vi "BenchC2.vi"() -> ()   [LabVIEW 2016]
uses:
  x64/Debug/BERTTA.dll
panel:
  out "element":bool
  out "Started:":string
  in  "SHUTDOWN":bool
  in  "MASTER CONTROL":bool
  in  "Tab Control":T1(tab)
  out "Output File":path caption="selected path"
  in  "Browse folder":path=path "" caption="start path"
  in  "Read Seq":bool
  in  "Save Seq":bool
  in  "Configuration file":path=path "C:/Users/shresplab/Desktop/ArttuConfiguration.lvm" caption="Filename"
  in  "OK Button 2":bool
  out "Boolean":bool
  in  "User (initials)":string
  in  "Project name":string
  in  "Description":string
  out "PUMP1":bool
  out "Target amount":dbl
  out "Scale weight":dbl
  out "Amount now":dbl
  out "Flow rate":dbl
  out "Time to target":dbl format="%<%H:%M:%S>t"
  out "Current step":dbl
  out "Target":dbl
  out "Amount now":dbl
  out "Amount now":dbl
  out "Target":dbl
  out "Current step":dbl
  out "Time to target":dbl format="%<%H:%M:%S>t"
  out "Flow rate":dbl
  out "Amount now":dbl
  out "Scale weight":dbl
  out "Target amount":dbl
  out "PUMP2":bool
  out "Sensor OK 6":bool
  out "Sensor OK 5":bool
  out "Sensor OK 4":bool
  out "Sensor OK 3":bool
  in  "OK Button":bool
  in  "Add comment":string
  out "PUMP3":bool
  out "Target amount":dbl
  out "Scale weight":dbl
  out "Amount now":dbl
  out "Flow rate":dbl
  out "Time to target":dbl format="%<%H:%M:%S>t"
  out "Current step":dbl
  out "Target":dbl
  out "Amount now":dbl
  out "Tr":dbl
  out "Tj in":dbl
  out "Tj out":dbl
  out "T set":dbl
  out "Current step":i32
  out "RPM":dbl
  out "Torque 2":dbl
  out "Waveform Chart 5":dynamicdata(graph)
  out "Waveform Chart 6":dynamicdata(graph)
  out "Waveform Chart 7":dynamicdata(graph)
  in  "Tab Control 2":T2(tab)
  out "Waveform Chart 3":dynamicdata(graph)
  out "Waveform Chart 8":dynamicdata(graph)
  out "Waveform Chart 11":dynamicdata(graph)
  out "Waveform Chart 13":dynamicdata(graph)
  out "Waveform Chart 9":dynamicdata(graph)
  out "Table":string[][](table)=[["14.8.2017 18.06.59", "0,000000", "417,670000", "-0,150000", "1,000000", "22,220000", "23,366837", "23,574959", "23,985852", "23,690000", "240,000000", "4,000000", "0,000000", "397,000000", "-397,000000", "1,000000"], ["14.8.2017 18.07.06", "0,000000", "417,640000", "-0,120000", "1,000000", "22,220000", "23,763115", "23,906257", "23,985694", "23,680000", "240,000000", "4,000000", "0,000000", "397,000000", "-397,000000", "1,000000"], ["14.8.2017 18.07.13", "0,000000", "417,640000", "-0,120000", "1,000000", "22,220000", "23,965922", "24,013440", "23,984906", "23,670000", "240,000000", "4,100000", "3,000000", "397,000000", "-397,000000", "1,000000"], ["14.8.2017 18.07.21", "0,000000", "417,640000", "-0,120000", "1,000000", "22,220000", "23,943860", "23,900110", "23,987113", "23,670000", "240,000000", "4,000000", "0,000000", "397,000000", "-397,000000", "1,000000"], ["14.8.2017 18.07.28", "0,000000", "417,640000", "-0,120000", "1,000000", "22,220000", "23,736328", "23,600018", "23,989004", "23,660000", "240,000000", "4,000000", "0,000000", "397,000000", "-397,000000", "1,000000"], ["14.8.2017 18.07.36", "0,000000", "417,640000", "-0,120000", "1,000000", "22,220000", "23,480910", "23,324538", "23,991053", "23,660000", "240,000000", "4,000000", "0,000000", "397,000000", "-397,000000", "1,000000"], ["14.8.2017 18.07.43", "0,000000", "417,640000", "-0,120000", "2,000000", "22,220000", "23,195579", "23,008270", "23,999093", "23,650000", "240,000000", "4,000000", "0,000000", "397,000000", "-397,000000", "1,000000"], ["14.8.2017 18.07.51", "0,000000", "417,650000", "-417,650000", "1,000000", "22,220000", "22,862541", "22,649021", "24,003979", "23,650000", "240,000000", "4,000000", "0,000000", "397,000000", "-397,000000", "2,000000"], ["14.8.2017 18.07.58", "0,000000", "417,640000", "0,010000", "1,000000", "22,220000", "22,541353", "22,354878", "24,005398", "23,650000", "240,000000", "4,000000", "0,000000", "397,000000", "-397,000000", "1,000000"], ["14.8.2017 18.08.06", "0,000000", "417,640000", "0,010000", "1,000000", "22,220000", "22,347931", "22,253738", "24,007605", "23,640000", "240,000000", "4,100000", "0,000000", "397,000000", "-397,000000", "1,000000"], ["14.8.2017 18.08.13", "0,000000", "417,640000", "0,010000", "1,000000", "22,220000", "22,329030", "22,302102", "24,006028", "23,640000", "240,000000", "4,000000", "0,000000", "395,820000", "-395,820000", "1,000000"], ["14.8.2017 18.08.20", "0,000000", "417,640000", "0,010000", "1,000000", "22,220000", "22,466849", "22,511320", "24,002403", "23,630000", "240,000000", "4,000000", "0,000000", "395,830000", "-0,010000", "1,000000"], ["14.8.2017 18.08.28", "0,000000", "417,640000", "0,010000", "1,000000", "22,220000", "22,707062", "22,835101", "24,000984", "23,620000", "240,000000", "4,000000", "0,000000", "395,830000", "-0,010000", "1,000000"], ["14.8.2017 18.08.35", "0,000000", "417,640000", "0,010000", "1,000000", "22,220000", "23,054104", "23,232979", "24,001299", "23,600000", "240,000000", "4,000000", "0,000000", "395,830000", "-0,010000", "1,000000"], ["14.8.2017 18.08.43", "0,000000", "417,640000", "0,010000", "1,000000", "22,220000", "23,412371", "23,522793", "24,002560", "23,590000", "240,000000", "4,000000", "0,000000", "395,820000", "0,000000", "1,000000"], ["14.8.2017 18.08.51", "0,000000", "417,640000", "0,010000", "1,000000", "22,220000", "23,596247", "23,656125", "24,003821", "23,580000", "240,000000", "4,000000", "0,000000", "395,820000", "0,000000", "1,000000"]]
  in  "X scale":i64(slide)=50 scale=0.0..100.0
  in  "Tr/Tj mode selector 2":bool=TRUE
  in  "Tr/Tj mode selector":bool=TRUE
  out "Boolean 4":bool
  out "Boolean 3":bool
  out "Boolean 2":bool
  in  "Reset 6":bool
  in  "Manual/Ramp":bool=TRUE
  in  "Array":dbl[][](array[numeric])=[[20.0, 0.0], [20.0, 0.0], [20.0, 0.0]]
  in  "?":bool
  in  "Time":dbl format="Time to target (min):                %#_g"
  out "Current temp":dbl format="Current temperature (S1):   %#_6g"
  in  "OK Button 3":bool
  out "Sensor OK":bool
  in  "T fail":dbl=20.0 format="Failsafe temperature:              %#_g"
  in  "Setpoint":dbl=20.0 format="Temperature target:                %#_6g"
  out "Waveform Chart":dynamicdata(graph)
  out "T external 2":dbl format="Current temp S2:    %#_g"
  in  "UPDATE TEMP":bool
  out "Led11 5":bool
  out "RPM":dbl format="%_4f"
  out "Led10 3":bool
  out "Led9 3":bool
  out "Led8 3":bool
  out "Led7 3":bool
  out "Led6 3":bool
  out "Led5 3":bool
  out "Led4 3":bool
  out "Led3 3":bool
  out "Led2 3":bool
  out "Led1 3":bool
  in  "PumpSeq 4":dbl[][](array[numeric])=[[0.0, 0.0, 0.0, 0.0, 0.0, 0.0, 0.0, 0.0, 0.0, 0.0], [0.0, 0.0, 0.0, 0.0, 0.0, 0.0, 0.0, 0.0, 0.0, 0.0], [0.0, 0.0, 0.0, 0.0, 0.0, 0.0, 0.0, 0.0, 0.0, 0.0], [0.0, 0.0, 0.0, 0.0, 0.0, 0.0, 0.0, 0.0, 0.0, 0.0], [0.0, 0.0, 0.0, 0.0, 0.0, 0.0, 0.0, 0.0, 0.0, 0.0], [0.0, 0.0, 0.0, 0.0, 0.0, 0.0, 0.0, 0.0, 0.0, 0.0], [0.0, 0.0, 0.0, 0.0, 0.0, 0.0, 0.0, 0.0, 0.0, 0.0], [0.0, 0.0, 0.0, 0.0, 0.0, 0.0, 0.0, 0.0, 0.0, 0.0], [0.0, 0.0, 0.0, 0.0, 0.0, 0.0, 0.0, 0.0, 0.0, 0.0], [0.0, 0.0, 0.0, 0.0, 0.0, 0.0, 0.0, 0.0, 0.0, 0.0]]
  in  "?":bool
  out "Flow rate (g/min)":dbl
  out "Scale reading":dbl
  out "Step amount now":dbl
  in  "Grams / min":dbl
  out "Waveform Chart 14":dynamicdata(graph)
  in  "?":bool
  out "Total amount now":dbl
  out "Led11 4":bool
  in  "Reset 5":bool
  out "Elapsed / step":i32
  out "Time to target":dbl format="%<%H:%M:%S>t"
  in  "OK Button 4":bool
  out "Led11":bool
  out "RPM":dbl format="%_4f"
  out "Led10":bool
  out "Led9":bool
  out "Led8":bool
  out "Led7":bool
  out "Led6":bool
  out "Led5":bool
  out "Led4":bool
  out "Led3":bool
  out "Led2":bool
  out "Led1":bool
  in  "PumpSeq 2":dbl[][](array[numeric])=[[0.0, 0.0, 0.0, 0.0, 0.0, 0.0, 0.0, 0.0, 0.0, 0.0], [0.0, 0.0, 0.0, 0.0, 0.0, 0.0, 0.0, 0.0, 0.0, 0.0], [0.0, 0.0, 0.0, 0.0, 0.0, 0.0, 0.0, 0.0, 0.0, 0.0], [0.0, 0.0, 0.0, 0.0, 0.0, 0.0, 0.0, 0.0, 0.0, 0.0], [0.0, 0.0, 0.0, 0.0, 0.0, 0.0, 0.0, 0.0, 0.0, 0.0], [0.0, 0.0, 0.0, 0.0, 0.0, 0.0, 0.0, 0.0, 0.0, 0.0], [0.0, 0.0, 0.0, 0.0, 0.0, 0.0, 0.0, 0.0, 0.0, 0.0], [0.0, 0.0, 0.0, 0.0, 0.0, 0.0, 0.0, 0.0, 0.0, 0.0], [0.0, 0.0, 0.0, 0.0, 0.0, 0.0, 0.0, 0.0, 0.0, 0.0], [0.0, 0.0, 0.0, 0.0, 0.0, 0.0, 0.0, 0.0, 0.0, 0.0]]
  in  "?":bool
  out "Flow rate (g/min)":dbl
  out "Scale reading":dbl
  out "Step amount now":dbl
  in  "Grams / min":dbl
  out "Waveform Chart 10":dynamicdata(graph)
  in  "?":bool
  out "Total amount now":dbl
  out "Led11":bool
  in  "Reset 3":bool
  out "Elapsed / step":i32
  out "Time to target":dbl format="%<%H:%M:%S>t"
  in  "OK Button 5":bool
  out "Led11 3":bool
  out "RPM":dbl format="%_4f"
  out "Led10 2":bool
  out "Led9 2":bool
  out "Led8 2":bool
  out "Led7 2":bool
  out "Led6 2":bool
  out "Led5 2":bool
  out "Led4 2":bool
  out "Led3 2":bool
  out "Led2 2":bool
  out "Led1 2":bool
  in  "PumpSeq 3":dbl[][](array[numeric])=[[0.0, 0.0, 0.0, 0.0, 0.0, 0.0, 0.0, 0.0, 0.0, 0.0], [0.0, 0.0, 0.0, 0.0, 0.0, 0.0, 0.0, 0.0, 0.0, 0.0], [0.0, 0.0, 0.0, 0.0, 0.0, 0.0, 0.0, 0.0, 0.0, 0.0], [0.0, 0.0, 0.0, 0.0, 0.0, 0.0, 0.0, 0.0, 0.0, 0.0], [0.0, 0.0, 0.0, 0.0, 0.0, 0.0, 0.0, 0.0, 0.0, 0.0], [0.0, 0.0, 0.0, 0.0, 0.0, 0.0, 0.0, 0.0, 0.0, 0.0], [0.0, 0.0, 0.0, 0.0, 0.0, 0.0, 0.0, 0.0, 0.0, 0.0], [0.0, 0.0, 0.0, 0.0, 0.0, 0.0, 0.0, 0.0, 0.0, 0.0], [0.0, 0.0, 0.0, 0.0, 0.0, 0.0, 0.0, 0.0, 0.0, 0.0], [0.0, 0.0, 0.0, 0.0, 0.0, 0.0, 0.0, 0.0, 0.0, 0.0]]
  in  "?":bool
  out "Flow rate (g/min)":dbl
  out "Scale reading":dbl
  out "Step amount now":dbl
  in  "Grams / min":dbl
  out "Waveform Chart 12":dynamicdata(graph)
  in  "?":bool
  out "Total amount now":dbl
  out "Led11 2":bool
  in  "Reset 4":bool
  out "Elapsed / step":i32
  out "Time to target":dbl format="%<%H:%M:%S>t"
  in  "OK Button 6":bool
  in  "?":bool
  in  "Scale port":dbl=5.0
  out "Waveform Chart 15":dynamicdata(graph)
  in  "?":bool
  in  "OK Button 8":bool
  in  "Remote / Manual":bool
  in  "Set RPM":i32
  out "RPM":dbl
  out "Torque":dbl
  out "Waveform Chart 4":dynamicdata(graph)
  in  "OK Button 7":bool
  out "PortDev out":dbl[](array[numeric])
  in  "Save PortDev":bool
  out "PortDev in":dbl[](array[numeric])
  in  "dev1":i32
  in  "dev2":i32
  in  "dev3":i32
  in  "dev4":i32
  in  "dev5":i32
  in  "dev6":i32
  in  "dev8":i32
  in  "port1":i32
  in  "port2":i32
  in  "port3":i32
  in  "port4":i32
  in  "port5":i32
  in  "port6":i32
  in  "port7":i32
  in  "port8":i32
  in  "dev7":i32
  in  "Treshold (T/C)":dbl=0.5
  out "DAQ 9217 (PT100)":errorcluster
  out "Config File":dbl[][](array[numeric])
  in  "Temp Control":tag="cDAQ9188XT-1C3BF2FMod1"
  in  "PAM Control":tag="cDAQ9188XT-1C3BF2FMod7"
  # "Temperature sensor:"
  # "Manual control:"
  # "PUMP & SCALE 1"
  # "STEP"
  # "TOTAL"
  # "PUMP & SCALE 2"
  # "STEP"
  # "TOTAL"
  # "PUMP & SCALE 3"
  # "STEP"
  # "TOTAL"
  # "Temperature control parameter"
  # "Secondary temperature sensor"
  # "Temp target"
  # "Time target"
  # "Grams    /   min"
  # "End of sequence"
  # "Manual control"
  # "Grams    /   min"
  # "End of sequence"
  # "Manual control"
  # "Grams    /   min"
  # "End of sequence"
  # "Manual control"
  # "PAM control"
  # "dev1 and dev2 always to port1 and 2\nport1 = port2 = Lauda\n\ndev3 and dev4 always to port3 and port4\nport3 = port4 = Heidolph"
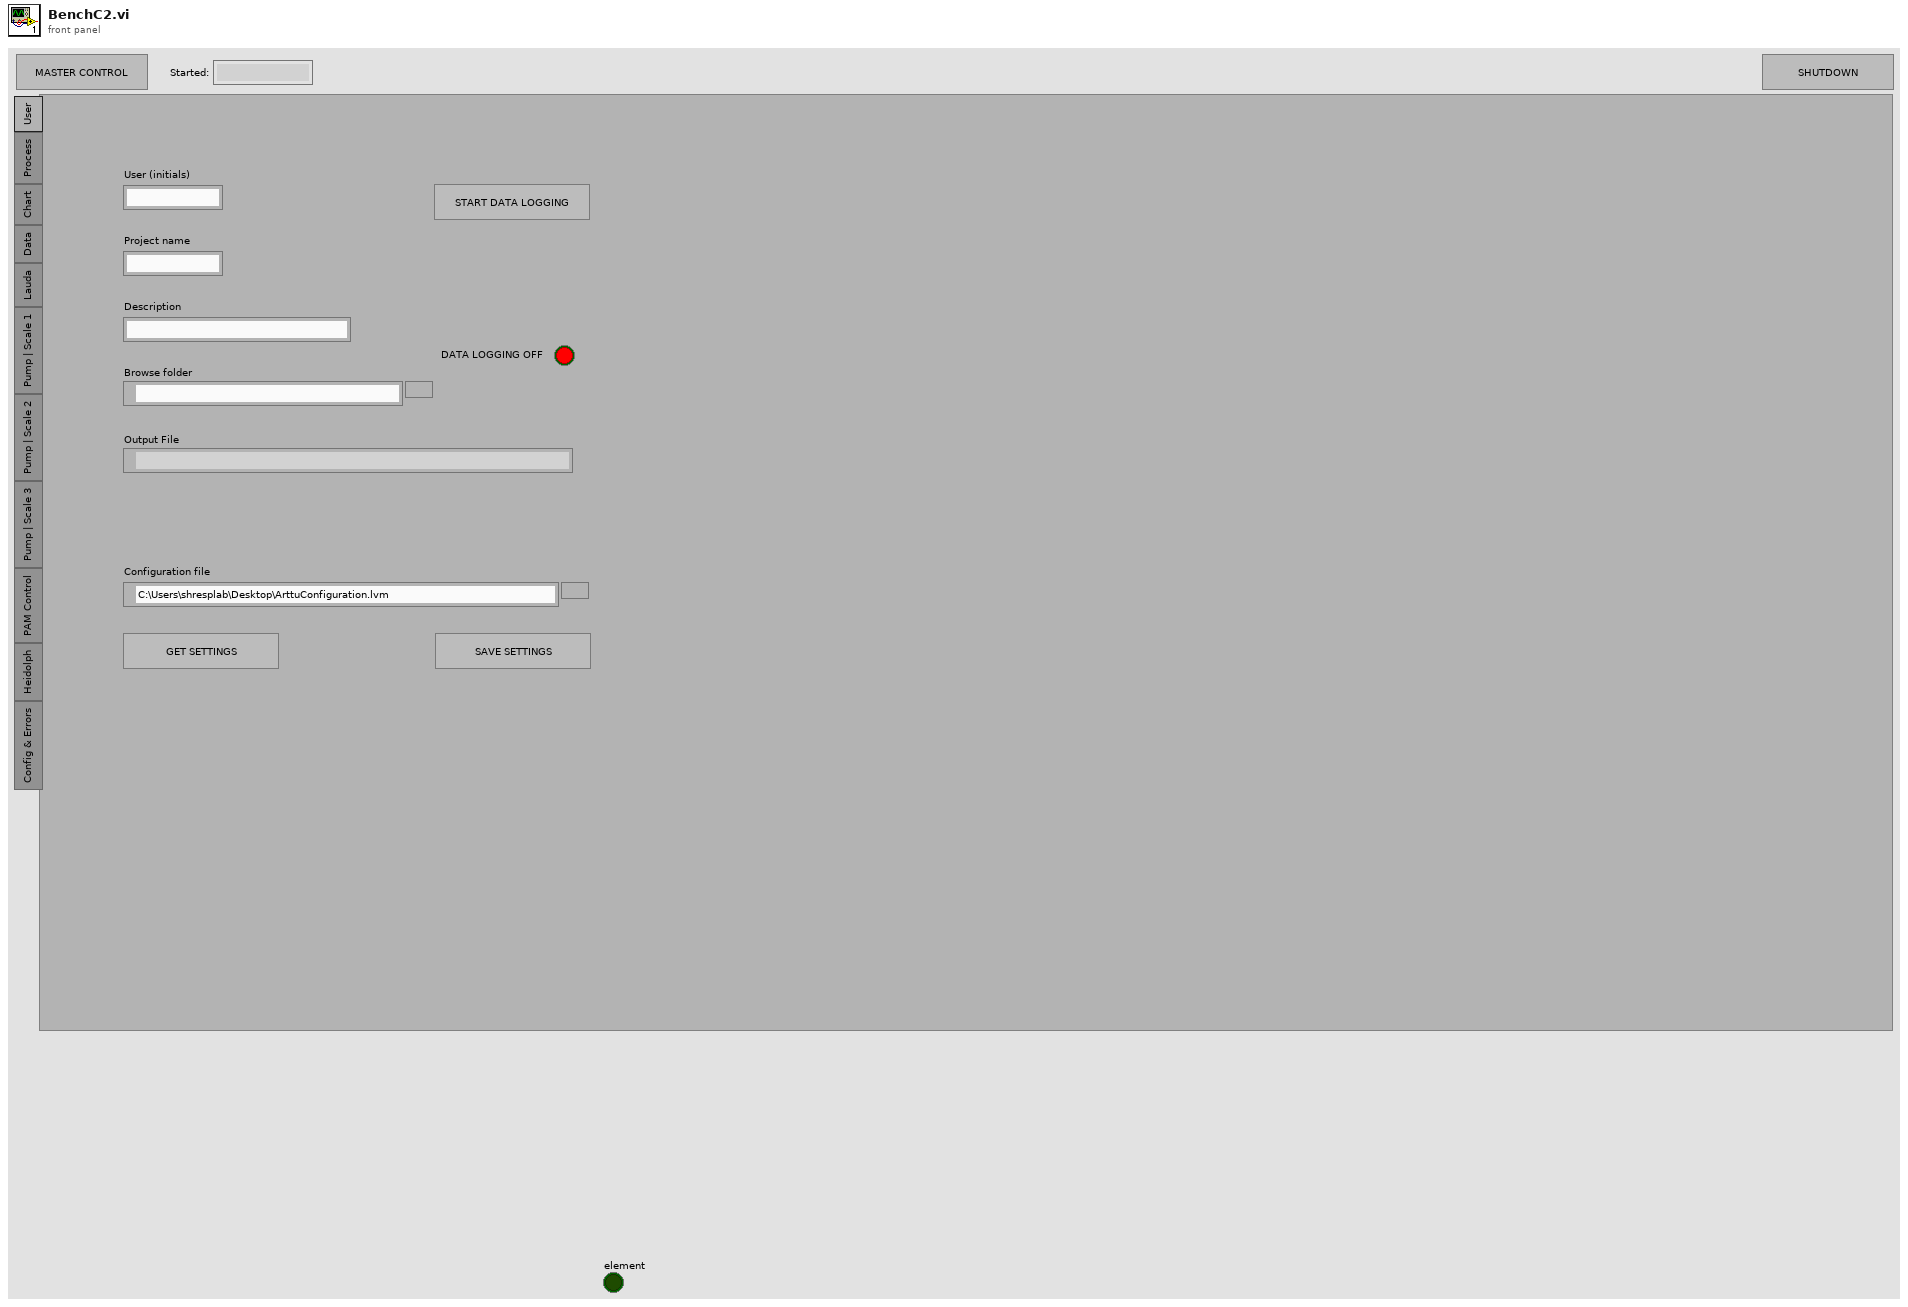
[diagram p1: front panel]
types:
  T1 = enum32{"User", "Process", "Chart", "Data", "Lauda", "Pump | Scale 1", "Pump | Scale 2", "Pump | Scale 3", "PAM Control", "Heidolph", "Config & Errors"}
  T2 = enum32{"Temperatures", "Scale / Pump 1", "Scale / Pump 2", "Scale / Pump 3", "RPM / torque"}
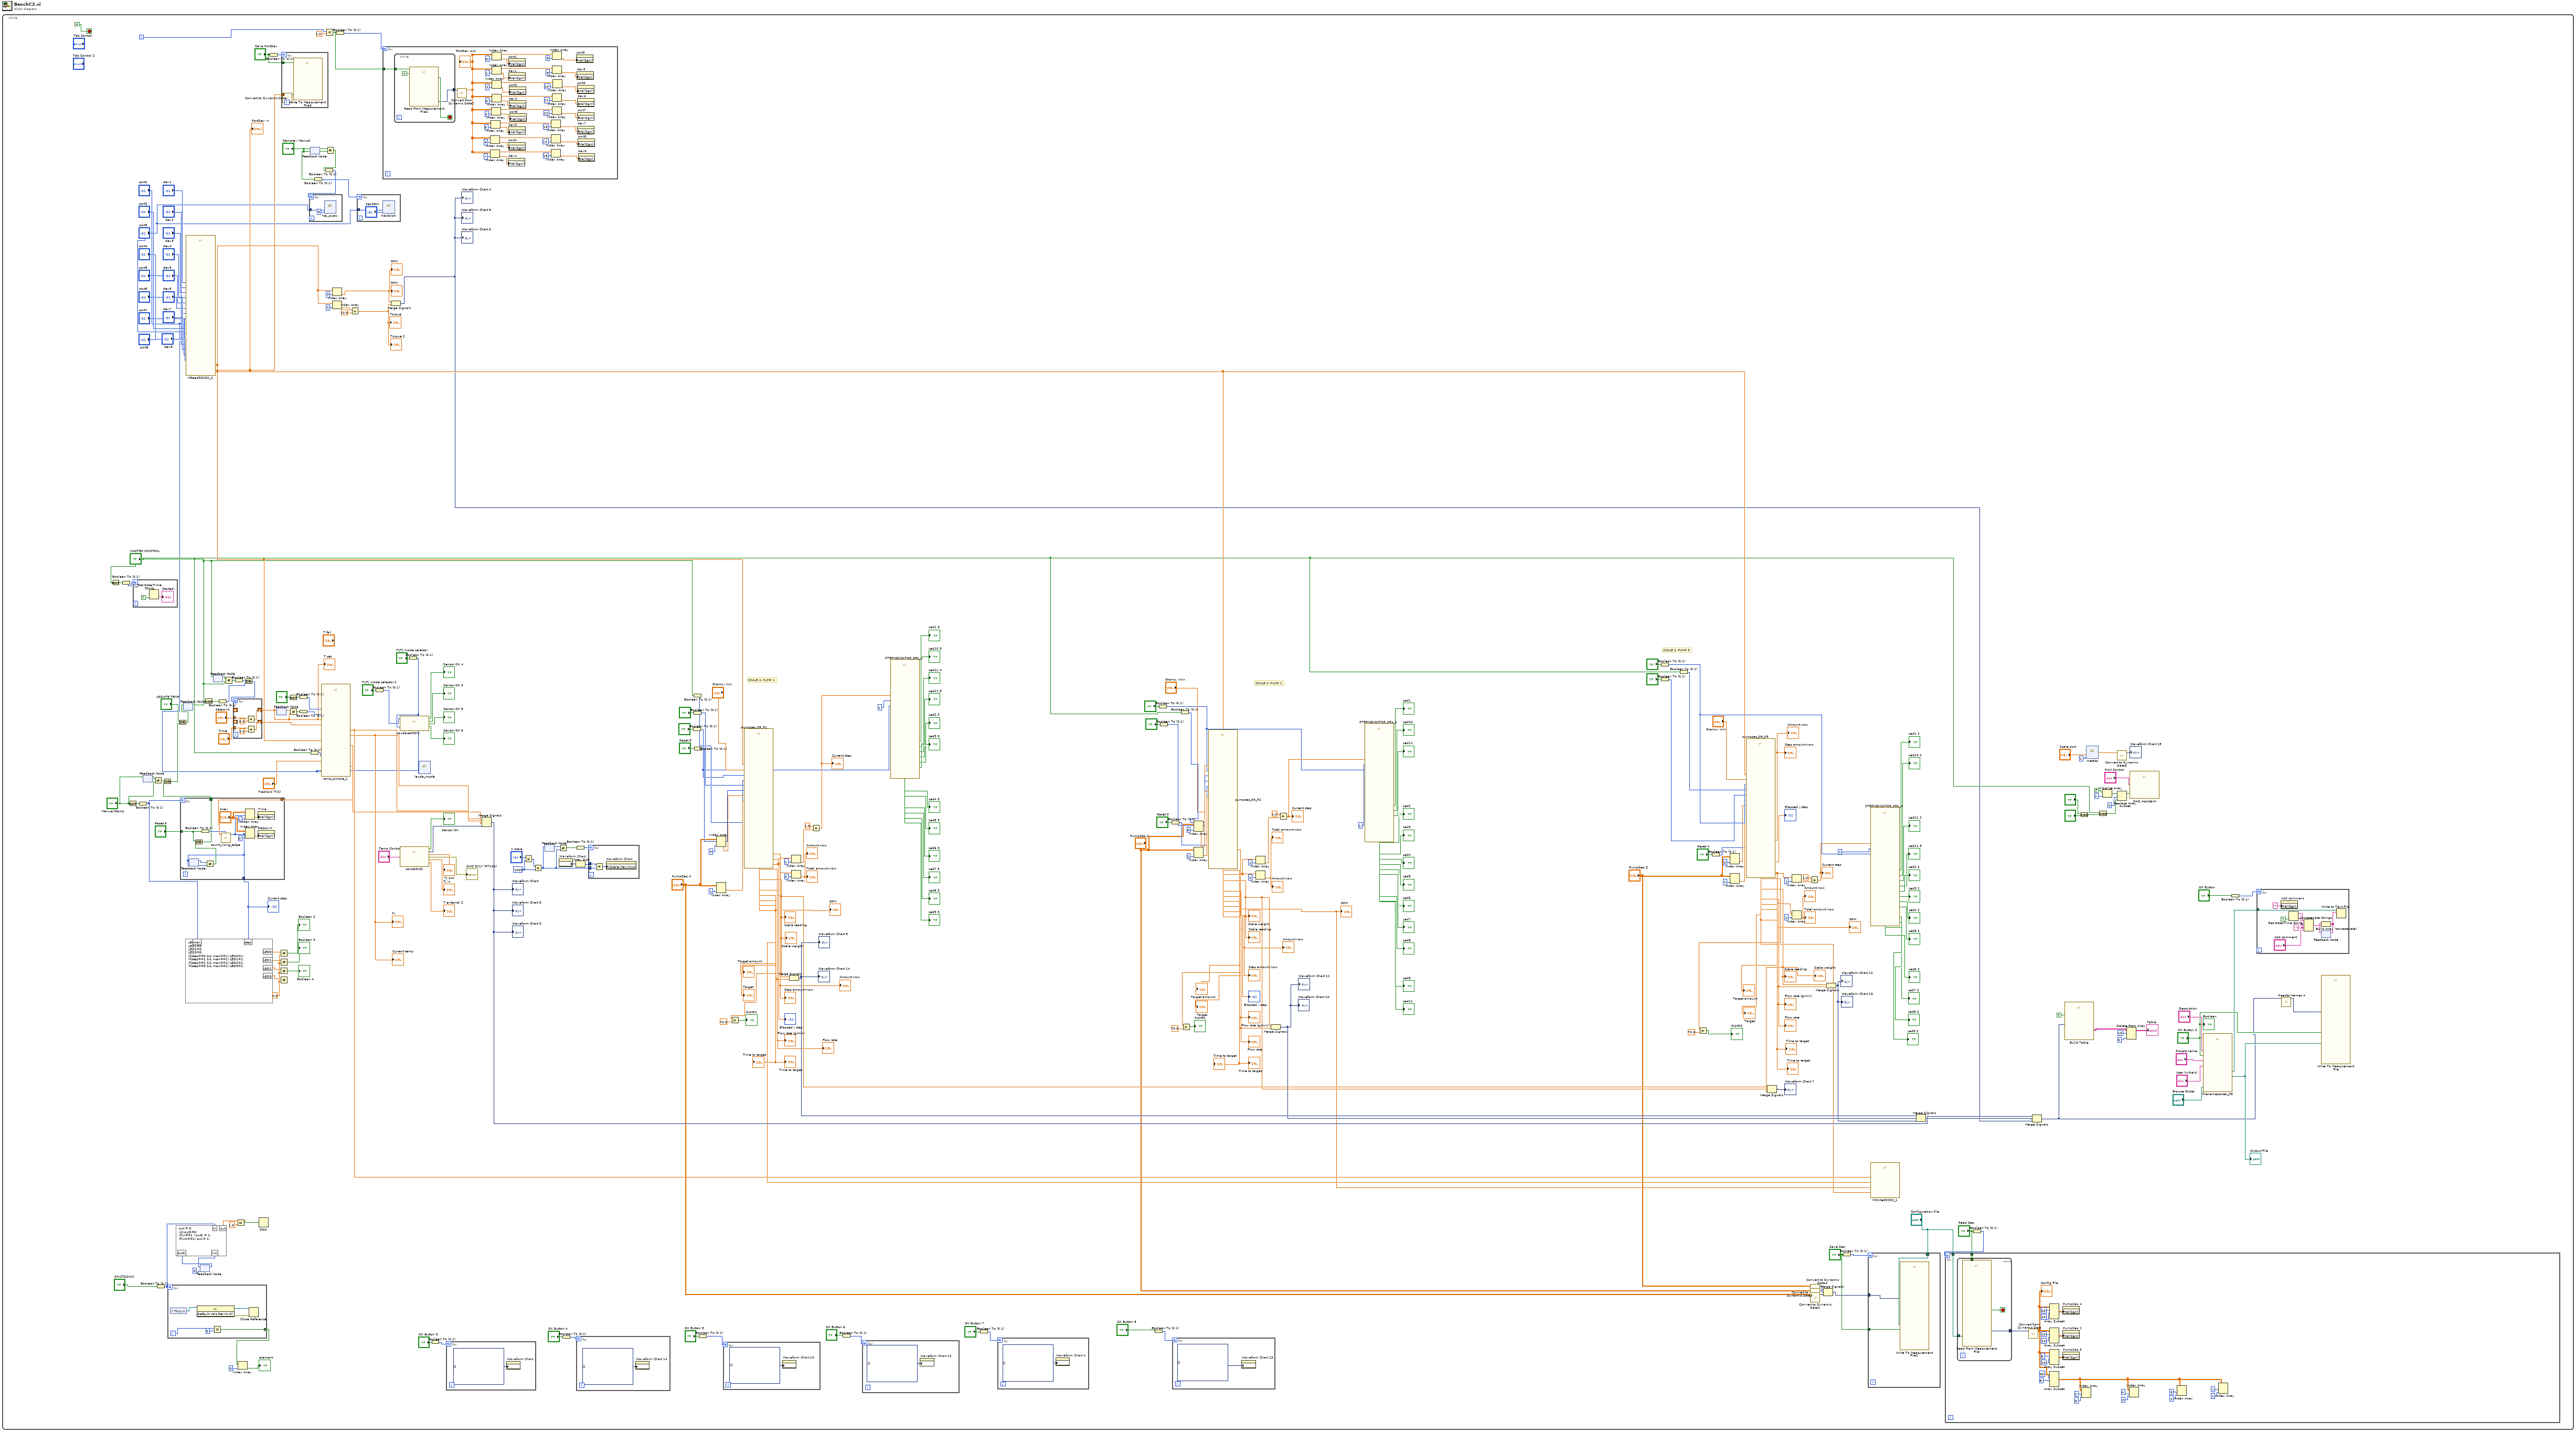
[diagram p0: block diagram]
diagram:
  n1 = while {
    i -> [w75]
    stop <- FALSE stop-if-true
    w6 = i64 1000 ("y")
    w61 = 0.0 ("y")
    # "SCALE & PUMP 1"
    # "SCALE & PUMP 3"
    # "SCALE & PUMP 2"
    n2 = Not(x="MASTER CONTROL") -> (.not. x?=w301:bool)
    n3 = Boolean To (0,1)(Boolean=w301) -> (0, 1=w302:i16)
    n4 = Not(x="Manual/Ramp") -> (.not. x?=w68:bool)
    n5 = for {
      N: w302 -> [_]
      n6 = Get Date/Time String(want seconds? (F)=TRUE) -> (time string=→"Started:":string)  [unwired: 2 in, 1 out]
    }
    n7 = Boolean To (0,1)(Boolean=w68) -> (0, 1=w51:i16)
    n8 = feedback #1() -> (w57:bool)  [unwired: 1 in]
    n9 = feedback-in #1("Manual/Ramp") -> ()
    n10 = Not Equal?(x=w57, y="Manual/Ramp") -> (x != y?=w54:bool)
    n11 = Boolean To (0,1)(Boolean="SHUTDOWN") -> (0, 1=w286:i16)
    n12 = for {
      N: w286 -> [_]
      tunnel: [w421] -> w300 mode=indexing
      i -> [w423]
      n13 = control-ref of="This VI"() -> (w426:refnum<vi>)
      n14 = invoke class="VI" method="Default Vals.Reinit All"(reference=w426) -> (reference out=w424:refnum<vi>, error out=w425:errorcluster)  [unwired: 2 in, 1 out]
      n15 = Greater?(x=w423, y=0) -> (0:w421:bool)
      n16 = Close Reference(reference=w424, error in (no error)=w425) -> ()  [unwired: 1 out]
    }
    n17 = feedback #2() -> (w49:bool)  [unwired: 1 in]
    n18 = call "MReadRS232_2.vi"("port1"="port1", "dev1"="dev1", "port2"="port2", "dev2"="dev2", "port3"="port3", "dev7"="dev7", "dev8"="dev8", "port7"="port7", "port8"="port8", "dev5"="dev5", "port5"="port5", "dev4"="dev4", "dev6"="dev6", "port6"="port6", "port4"="port4", "dev3"="dev3") -> ("output array"=w79:dbl[], "params"=w41:dbl[])  [unwired: 2 in]
    "PortDev in" <- w79
    n19 = feedback #3(0) -> (w284:i32)
    n20 = formula code="out = 0;\nint out2=0;\nif(in==1 ) out2 = 1;\nif(in2==1) out = 1;"("in"=w286, "in2"=w284) -> ("out"=w288:dbl, "out2"=w285:i32)
    n21 = feedback-in #3(w285) -> ()
    n22 = And(x="MASTER CONTROL", y=w49) -> (x .and. y?=w105:bool)
    n23 = feedback #4() -> (w97:bool)  [unwired: 1 in]
    n24 = feedback-in #4("MASTER CONTROL") -> ()
    n25 = Boolean To (0,1)(Boolean=w105) -> (0, 1=w95:i16)
    n26 = Not Equal?(x=w97, y="MASTER CONTROL") -> (x != y?=w96:bool)
    n27 = Boolean To (0,1)(Boolean=w96) -> (0, 1=w94:i16)
    n28 = Equal?(x=w288, y=1.0) -> (x = y?=w287:bool)
    n29 = Index Array(array=w300, index=0) -> (element=→"element":bool)
    n30 = Or(x=w94, y=w95) -> (x .or. y?=w93:i16)
    n31 = for {
      N: w93 -> [_]
      tunnel: "Time" -> [w373]
      shift-right: [w372] -> w106
      shift-left: _ -> [_]
      tunnel: "Setpoint" -> [w370]
      shift-right: [w369] -> w15
      shift-left: _ -> [_]
      n32 = Add(x=w370, y=0.0) -> (x+y=w369:dbl)
      n33 = Add(x=w373, y=0.0) -> (x+y=w372:dbl)
    }
    "T set" <- w15
    n34 = Stop(stop? (T)=w287) -> ()
    n35 = Boolean To (0,1)(Boolean="Save PortDev") -> (0, 1=w78:i16)
    n36 = feedback-in #5(w15) -> ()
    n37 = feedback #5() -> (w104:dbl)  [unwired: 1 in]
    n38 = for {
      N: w78 -> [_]
      tunnel: w79 -> [w368]
      tunnel: "Save PortDev" -> [w366]
      n39 = call "Convert to Dynamic Data"("Array"=w368) -> ("Dynamic Data Type"=w367:dynamicdata)  [unwired: 3 in]
      n40 = call "Write To Measurement File3"("Signals"=w367, "Reset"=w366) -> ()  [unwired: 15 in, 3 out]
    }
    n41 = Not(x="?") -> (.not. x?=w100:bool)
    n42 = Not Equal?(x=w104, y=w15) -> (x != y?=w103:bool)
    n43 = Boolean To (0,1)(Boolean=w100) -> (0, 1=w102:i16)
    n44 = Boolean To (0,1)(Boolean=w103) -> (0, 1=w98:i16)
    n45 = Boolean To (0,1)(Boolean="MASTER CONTROL") -> (0, 1=w99:i16)
    n46 = feedback-in #6("Remote / Manual") -> ()
    n47 = feedback #6() -> (w46:bool)  [unwired: 1 in]
    n48 = Boolean To (0,1)(Boolean="Remote / Manual") -> (0, 1=w44:i16)
    n49 = call "ramp_simple_1.vi"("pause"=w102, "time_set"=w106, "array"=w41, "reset"=w98, "master"=w99, "T_sp"=w15, "treshold"="Treshold (T/C)", "port"="port1") -> ("Tin"=w109:dbl, "Tr"=w110:dbl, "target_reached"=w66:dbl, "T control"=w111:dbl)  [unwired: 3 in, 1 out]
    "Tr" <- w110
    "Current temp" <- w110
    n50 = for {
      N: w51 -> [_]
      tunnel: w66 -> [w325]
      tunnel: [w315] -> w55
      tunnel: "Reset 6" -> [w317]
      tunnel: [w318] -> w16
      n51 = feedback #7() -> (w319:i32)  [unwired: 1 in]
      n52 = Boolean To (0,1)(Boolean=w317) -> (0, 1=w320:i16)
      n53 = call "count_rising_edge.vi"("reset"=w320, "target_reached"=w325) -> ("element 2"=w318:i32)  [unwired: 9 in]
      n54 = feedback-in #7(w318) -> ()
      n55 = Not Equal?(x=w319, y=w318) -> (x != y?=w316:bool)
      n56 = Or(x=w317, y=w316) -> (x .or. y?=w315:bool)
      n57 = Index Array(array="Array", index (row)=w318, index (col)=1 ("disabled index (col)")) -> (element=w321:dbl)
      n58 = Index Array(array="Array", index (row)=w318, index (col)=0 ("disabled index (col)")) -> (element=w322:dbl)
      n59 = property on="Time" class="DigNum (strict)"("Val(Sgnl)"=w321) -> ()  [unwired: 2 in, 2 out]
      n60 = property on="Setpoint" class="DigNum (strict)"("Val(Sgnl)"=w322) -> ()  [unwired: 2 in, 2 out]
    }
    "Current step" <- w16
    n61 = Or(x=w54, y=w55) -> (x .or. y?=w53:bool)
    n62 = Or(x="UPDATE TEMP", y=w53) -> (x .or. y?=w50:bool)
    n63 = feedback-in #2(w50) -> ()
    n64 = formula code="LED0=0;\nLED1=0;\nLED2=0;\nLED3=0;\nif(step==0 && man==1) LED0=1;\nif(step==1 && man==1) LED1=1;\nif(step==2 && man==1) LED2=1;\nif(step==3 && man==1) LED3=1;"("step"=w16, "man"=w51) -> ("LED0"=w65:dbl, "LED1"=w64:dbl, "LED2"=w63:dbl, "LED3"=w62:dbl)
    n65 = Not Equal?(x=w65, y=w61) -> (x != y?=→"Boolean 2":bool)
    n66 = Not Equal?(x=w64, y=w61) -> (x != y?=→"Boolean 3":bool)
    n67 = Not Equal?(x=w63, y=w61) -> (x != y?=→"Boolean 4":bool)
    n68 = Not Equal?(x=w62, y=w61) -> ()  [unwired: 1 out]
    n69 = Less?(x=w75, y=1.0) -> (x < y?=w73:bool)
    n70 = Not Equal?(x=w46, y="Remote / Manual") -> (x != y?=w45:bool)
    n71 = Boolean To (0,1)(Boolean=w45) -> (0, 1=w47:i16)
    n72 = for {
      N: w47 -> [_]
      tunnel: "port3" -> [w313]
      n73 = dll-call lib="C:/Users/shresplab/OneDrive - Kemira Oyj/Documents/GitHub/Bertta/BERTTA/x64/Debug/BERTTA.dll" fn="hei_query"("port"=w313, "q"=5) -> ()  [unwired: 6 in, 2 out]
    }
    n74 = Index Array(array=w41, index=3) -> (element=w38:dbl)
    "RPM" <- w38
    "RPM" <- w38
    n75 = Index Array(array=w41, index=2) -> (element=w40:dbl)
    n76 = Boolean To (0,1)(Boolean=w73) -> (0, 1=w74:i16)
    n77 = Divide(x=w40, y=10.0) -> (x/y=w37:dbl)
    "Torque" <- w37
    "Torque 2" <- w37
    n78 = for {
      N: w44 -> [_]
      tunnel: "port3" -> [w311]
      n79 = dll-call lib="C:/Users/shresplab/OneDrive - Kemira Oyj/Documents/GitHub/Bertta/BERTTA/x64/Debug/BERTTA.dll" fn="heidolph"("port"=w311, "speed"="Set RPM") -> ()  [unwired: 6 in, 2 out]
    }
    n80 = Boolean To (0,1)(Boolean="Tr/Tj mode selector 2") -> (0, 1=w10:i16)
    n81 = for {
      N: w74 -> [_]
      tunnel: w73 -> [w361]
      n82 = while {
        tunnel: [w364] -> w360
        tunnel: w361 -> [w362]
        stop <- w365 stop-if-true
        n83 = call "Read From Measurement File2"("Enable"=TRUE, "Reset"=w362) -> ("Signals"=w364:dynamicdata, "EOF?"=w365:bool)  [unwired: 4 in, 4 out]
      }
      n84 = call "Convert from Dynamic Data2"("Dynamic Data Type"=w360) -> ("Array"=w343:dbl[])  [unwired: 3 in]
      "PortDev out" <- w343
      n85 = Index Array(array=w343, index=6) -> (element=w336:dbl)
      n86 = Index Array(array=w343, index=7) -> (element=w335:dbl)
      n87 = Index Array(array=w343, index=5) -> (element=w337:dbl)
      n88 = Index Array(array=w343, index=4) -> (element=w338:dbl)
      n89 = Index Array(array=w343, index=0) -> (element=w342:dbl)
      n90 = Index Array(array=w343, index=1) -> (element=w341:dbl)
      n91 = Index Array(array=w343, index=3) -> (element=w339:dbl)
      n92 = Index Array(array=w343, index=2) -> (element=w340:dbl)
      n93 = property on="dev4" class="DigNum (strict)"("Val(Sgnl)"=w335) -> ()  [unwired: 2 in, 2 out]
      n94 = property on="dev3" class="DigNum (strict)"("Val(Sgnl)"=w337) -> ()  [unwired: 2 in, 2 out]
      n95 = property on="port4" class="DigNum (strict)"("Val(Sgnl)"=w336) -> ()  [unwired: 2 in, 2 out]
      n96 = property on="port1" class="DigNum (strict)"("Val(Sgnl)"=w342) -> ()  [unwired: 2 in, 2 out]
      n97 = property on="dev1" class="DigNum (strict)"("Val(Sgnl)"=w341) -> ()  [unwired: 2 in, 2 out]
      n98 = property on="port2" class="DigNum (strict)"("Val(Sgnl)"=w340) -> ()  [unwired: 2 in, 2 out]
      n99 = property on="dev2" class="DigNum (strict)"("Val(Sgnl)"=w339) -> ()  [unwired: 2 in, 2 out]
      n100 = property on="port3" class="DigNum (strict)"("Val(Sgnl)"=w338) -> ()  [unwired: 2 in, 2 out]
      n101 = Index Array(array=w343, index=14) -> (element=w328:dbl)
      n102 = Index Array(array=w343, index=15) -> (element=w327:dbl)
      n103 = Index Array(array=w343, index=13) -> (element=w329:dbl)
      n104 = Index Array(array=w343, index=12) -> (element=w330:dbl)
      n105 = Index Array(array=w343, index=8) -> (element=w334:dbl)
      n106 = Index Array(array=w343, index=9) -> (element=w333:dbl)
      n107 = Index Array(array=w343, index=11) -> (element=w331:dbl)
      n108 = Index Array(array=w343, index=10) -> (element=w332:dbl)
      n109 = property on="port5" class="DigNum (strict)"("Val(Sgnl)"=w334) -> ()  [unwired: 2 in, 2 out]
      n110 = property on="dev5" class="DigNum (strict)"("Val(Sgnl)"=w333) -> ()  [unwired: 2 in, 2 out]
      n111 = property on="port6" class="DigNum (strict)"("Val(Sgnl)"=w332) -> ()  [unwired: 2 in, 2 out]
      n112 = property on="dev6" class="DigNum (strict)"("Val(Sgnl)"=w331) -> ()  [unwired: 2 in, 2 out]
      n113 = property on="port7" class="DigNum (strict)"("Val(Sgnl)"=w330) -> ()  [unwired: 2 in, 2 out]
      n114 = property on="dev7" class="DigNum (strict)"("Val(Sgnl)"=w329) -> ()  [unwired: 2 in, 2 out]
      n115 = property on="port8" class="DigNum (strict)"("Val(Sgnl)"=w328) -> ()  [unwired: 2 in, 2 out]
      n116 = property on="dev8" class="DigNum (strict)"("Val(Sgnl)"=w327) -> ()  [unwired: 2 in, 2 out]
    }
    n117 = Merge Signals(w38, w37) -> (w36:dynamicdata)
    "Waveform Chart 4" <- w36
    "Waveform Chart 6" <- w36
    "Waveform Chart 9" <- w36
    n118 = call "LaudaDAQ.vi"("device name"="Temp Control") -> ("error out"=→"DAQ 9217 (PT100)":errorcluster, 1:"Tj out"=→"Tj out":dbl, "data"=w178:dynamicdata, "Sensor OK"=→"Sensor OK":bool, 4:"Tj out"=→"Tj in":dbl, "T external 2"=→"T external 2":dbl)  [unwired: 5 in]
    n119 = Boolean To (0,1)(Boolean="Tr/Tj mode selector") -> (0, 1=w12:i16)
    n120 = call "LaudaLedCtrl2.vi"("ctrl_mode"=w12, "T ext / T ext in"=w10) -> ("Sensor OK 5"=→"Sensor OK 5":bool, "Sensor OK 3"=→"Sensor OK 3":bool, "Sensor OK 4"=→"Sensor OK 4":bool, "Sensor OK 6"=→"Sensor OK 6":bool)  [unwired: 6 in]
    n121 = dll-call lib="C:/Users/shresplab/OneDrive - Kemira Oyj/Documents/GitHub/Bertta/BERTTA/x64/Debug/BERTTA.dll" fn="lauda_mode"("port"="port1", "mode"=w12) -> ()  [unwired: 6 in, 2 out]
    n122 = Boolean To (0,1)(Boolean="OK Button 3") -> (0, 1=w122:i16)
    n123 = for {
      N: w122 -> [_]
      n124 = property on="Waveform Chart" class="WFChart (strict)"("History Data"=dynamicdata[] []) -> ()  [unwired: 2 in, 2 out]
    }
    n125 = Merge Signals(w111, w110, w109, w178) -> (w179:dynamicdata)
    "Waveform Chart 3" <- w179
    "Waveform Chart" <- w179
    "Waveform Chart 5" <- w179
    n126 = Multiply(x="X scale", y=w6) -> (x*y=w7:i64)
    n127 = Add(x=w7, y=w6) -> (x+y=w2:i64)
    n128 = feedback-in #8(w2) -> ()
    n129 = feedback #8() -> (w5:i64)  [unwired: 1 in]
    n130 = Not Equal?(x=w5, y=w2) -> (x != y?=w4:bool)
    n131 = property on="Waveform Chart" class="WFChart (strict)"() -> ("History Data"=w9:dynamicdata[])  [unwired: 2 in, 2 out]
    n132 = Boolean To (0,1)(Boolean="OK Button 4") -> (0, 1=w120:i16)
    n133 = Boolean To (0,1)(Boolean=w4) -> (0, 1=w1:i16)
    n134 = Array Size(array=w9) -> (size(s)=w3:i32)
    n135 = for {
      N: w120 -> [_]
      n136 = property on="Waveform Chart 14" class="WFChart (strict)"("History Data"=dynamicdata[] []) -> ()  [unwired: 2 in, 2 out]
    }
    n137 = for {
      N: w1 -> [_]
      tunnel: w3 -> [w309]
      tunnel: w2 -> [w308]
      n138 = Add(x=w309, y=w308) -> (x+y=w307:i64)
      n139 = property on="Waveform Chart" class="WFChart (strict)"("XScale.Maximum"=w307) -> ()  [unwired: 2 in, 2 out]
    }
    n140 = Boolean To (0,1)(Boolean="?") -> (0, 1=w187:i16)
    n141 = Boolean To (0,1)(Boolean="?") -> (0, 1=w191:i16)
    n142 = Boolean To (0,1)(Boolean="MASTER CONTROL") -> (0, 1=w183:i16)
    n143 = Boolean To (0,1)(Boolean="Reset 5") -> (0, 1=w190:i16)
    n144 = Boolean To (0,1)(Boolean="OK Button 5") -> (0, 1=w118:i16)
    n145 = Index Array(array="PumpSeq 4", index (col)=0) -> (element=w195:dbl[])  [unwired: 1 in]
    n146 = Index Array(array="PumpSeq 4", index (col)=1) -> (element=w216:dbl[])  [unwired: 1 in]
    n147 = for {
      N: w118 -> [_]
      n148 = property on="Waveform Chart 10" class="WFChart (strict)"("History Data"=dynamicdata[] []) -> ()  [unwired: 2 in, 2 out]
    }
    n149 = call "pumpsec_09_P1.vi"("reset"=w190, "master"=w183, "manual"=w187, "pause"=w191, "Array"=w41, "Target"=w195, "fr_manual"="Grams / min", "Time"=w216) -> ("pumpCtrl"=w162:dbl, "totaltarget"=→"Target":dbl, "target_step"=→"Target amount":dbl, "REGLO D"=w128:dbl, "time_to_target"=→"Time to target" →"Time to target":dbl, "step_fr"=w139:dbl, "amount_step"=→"Amount now" →"Step amount now":dbl, "Scale"=w174:dbl, "elapsed_step"=→"Elapsed / step":dbl, "params"=w213:dbl[])  [unwired: 8 in, 2 out]
    "Flow rate" <- w139
    "Scale weight" <- w174
    "Scale reading" <- w174
    "Flow rate (g/min)" <- w139
    "RPM" <- w128
    n150 = Greater?(x=w162, y=70.0) -> (0:→"PUMP1":bool)
    n151 = Merge Signals(w174, w139) -> (w182:dynamicdata)
    "Waveform Chart 8" <- w182
    "Waveform Chart 14" <- w182
    n152 = Index Array(array=w213, index=1) -> (element=w210:dbl)
    n153 = Index Array(array=w213, index=2) -> (element=→"Amount now" →"Total amount now":dbl)
    n154 = Add(x=1.0, y=w210) -> (x+y=w140:dbl)
    "Current step" <- w140
    n155 = Boolean To (0,1)(Boolean="OK Button 6") -> (0, 1=w116:i16)
    n156 = for {
      N: w116 -> [_]
      n157 = property on="Waveform Chart 12" class="WFChart (strict)"("History Data"=dynamicdata[] []) -> ()  [unwired: 2 in, 2 out]
    }
    n158 = call "STEPINDICATOR_091_2.vi"("current step"=w140, "enable"=i16 1, "manual"=w187) -> ("Led 8"=→"Led8 3":bool, "Led 10"=→"Led10 3":bool, "Led 11"=→"Led11 4":bool, "Led 7"=→"Led7 3":bool, "Led 1"=→"Led1 3":bool, "Led 6"=→"Led6 3":bool, "Led 2"=→"Led2 3":bool, "Led 12"=→"Led11 5":bool, "Led 5"=→"Led5 3":bool, "Led 4"=→"Led4 3":bool, "Led 3"=→"Led3 3":bool, "Led 9"=→"Led9 3":bool)  [unwired: 1 in]
    n159 = Boolean To (0,1)(Boolean="OK Button 7") -> (0, 1=w114:i16)
    n160 = for {
      N: w114 -> [_]
      n161 = property on="Waveform Chart 4" class="WFChart (strict)"("History Data"=dynamicdata[] []) -> ()  [unwired: 2 in, 2 out]
    }
    n162 = Boolean To (0,1)(Boolean="OK Button 8") -> (0, 1=w33:i16)
    n163 = Boolean To (0,1)(Boolean="?") -> (0, 1=w250:i16)
    n164 = Boolean To (0,1)(Boolean="?") -> (0, 1=w276:i16)
    n165 = Boolean To (0,1)(Boolean="Reset 3") -> (0, 1=w274:i16)
    n166 = for {
      N: w33 -> [_]
      n167 = property on="Waveform Chart 15" class="WFChart (strict)"("History Data"=dynamicdata[] []) -> ()  [unwired: 2 in, 2 out]
    }
    n168 = Boolean To (0,1)(Boolean="MASTER CONTROL") -> (0, 1=w268:i16)
    n169 = Index Array(array="PumpSeq 2", index (col)=0 ("disabled index (col)")) -> (element=w279:dbl[])  [unwired: 1 in]
    n170 = Index Array(array="PumpSeq 2", index (col)=1 ("disabled index (col)")) -> (element=w278:dbl[])  [unwired: 1 in]
    n171 = call "pumpsec_09_P2.vi"("reset"=w274, "master"=w268, "manual"=w250, "pause"=w276, "Array"=w41, "Target"=w279, "fr_manual"="Grams / min", "Time"=w278) -> ("pumpCtrl"=w158:dbl, "totaltarget"=→"Target":dbl, "target_step"=→"Target amount":dbl, "REGLO D"=w127:dbl, "time_to_target"=→"Time to target" →"Time to target":dbl, "step_fr"=w177:dbl, "amount_step"=→"Amount now" →"Step amount now":dbl, "Scale"=w173:dbl, "elapsed_step"=→"Elapsed / step":dbl, "params"=w269:dbl[])  [unwired: 8 in, 2 out]
    "Scale weight" <- w173
    "Flow rate" <- w177
    "Scale reading" <- w173
    "Flow rate (g/min)" <- w177
    "RPM" <- w127
    n172 = Greater?(x=w158, y=70.0) -> (0:→"PUMP2":bool)
    n173 = Index Array(array=w269, index=1) -> (element=w272:dbl)
    n174 = Index Array(array=w269, index=2) -> (element=→"Amount now" →"Total amount now":dbl)
    n175 = Merge Signals(w173, w177) -> (w184:dynamicdata)
    "Waveform Chart 11" <- w184
    "Waveform Chart 10" <- w184
    n176 = Add(x=1.0, y=w272) -> (x+y=w266:dbl)
    "Current step" <- w266
    n177 = call "STEPINDICATOR_091_2.vi"("current step"=w266, "enable"=i16 1, "manual"=w250) -> ("Led 8"=→"Led8":bool, "Led 10"=→"Led10":bool, "Led 11"=→"Led11":bool, "Led 7"=→"Led7":bool, "Led 1"=→"Led1":bool, "Led 6"=→"Led6":bool, "Led 2"=→"Led2":bool, "Led 12"=→"Led11":bool, "Led 5"=→"Led5":bool, "Led 4"=→"Led4":bool, "Led 3"=→"Led3":bool, "Led 9"=→"Led9":bool)  [unwired: 1 in]
    n178 = Boolean To (0,1)(Boolean="?") -> (0, 1=w244:i16)
    n179 = Boolean To (0,1)(Boolean="?") -> (0, 1=w243:i16)
    n180 = Boolean To (0,1)(Boolean="MASTER CONTROL") -> (0, 1=w245:i16)
    n181 = Boolean To (0,1)(Boolean="Reset 4") -> (0, 1=w225:i16)
    n182 = Index Array(array="PumpSeq 3", index (col)=0 ("disabled index (col)")) -> (element=w228:dbl[])  [unwired: 1 in]
    n183 = Index Array(array="PumpSeq 3", index (col)=1 ("disabled index (col)")) -> (element=w227:dbl[])  [unwired: 1 in]
    n184 = call "pumpsec_09_P3.vi"("reset"=w225, "master"=w245, "manual"=w244, "pause"=w243, "Array"=w41, "Target"=w228, "fr_manual"="Grams / min", "Time"=w227) -> ("pumpCtrl"=w155:dbl, "totaltarget"=→"Target":dbl, "target_step"=→"Target amount":dbl, "REGLO D"=w126:dbl, "time_to_target"=→"Time to target" →"Time to target":dbl, "step_fr"=w176:dbl, "amount_step"=→"Amount now" →"Step amount now":dbl, "Scale"=w172:dbl, "elapsed_step"=→"Elapsed / step":dbl, "params"=w218:dbl[])  [unwired: 8 in, 2 out]
    "Scale weight" <- w172
    "Flow rate" <- w176
    "Scale reading" <- w172
    "Flow rate (g/min)" <- w176
    "RPM" <- w126
    n185 = Greater?(x=w155, y=70.0) -> (0:→"PUMP3":bool)
    n186 = Merge Signals(w174, w173, w172) -> (→"Waveform Chart 7":dynamicdata)
    n187 = Index Array(array=w218, index=1) -> (element=w219:dbl)
    n188 = Index Array(array=w218, index=2) -> (element=→"Amount now" →"Total amount now":dbl)
    n189 = Add(x=1.0, y=w219) -> (x+y=w217:dbl)
    "Current step" <- w217
    n190 = call "Convert to Dynamic Data4"("2D Array"="PumpSeq 3") -> ("Dynamic Data Type"=w131:dynamicdata)  [unwired: 3 in]
    n191 = call "Convert to Dynamic Data3"("2D Array"="PumpSeq 2") -> ("Dynamic Data Type"=w133:dynamicdata)  [unwired: 3 in]
    n192 = call "Convert to Dynamic Data2"("2D Array"="PumpSeq 4") -> ("Dynamic Data Type"=w136:dynamicdata)  [unwired: 3 in]
    n193 = Merge Signals(w131, w133, w136) -> (w135:dynamicdata)
    n194 = Merge Signals(w172, w176) -> (w181:dynamicdata)
    "Waveform Chart 13" <- w181
    "Waveform Chart 12" <- w181
    n195 = Boolean To (0,1)(Boolean="Save Seq") -> (0, 1=w130:i16)
    n196 = for {
      N: w130 -> [_]
      tunnel: w135 -> [w419]
      tunnel: "Configuration file" -> [w420]
      tunnel: "Save Seq" -> [w418]
      n197 = call "Write To Measurement File2"("Signals"=w419, "Reset"=w418, "Filename"=w420) -> ()  [unwired: 14 in, 3 out]
    }
    n198 = call "STEPINDICATOR_091_4.vi"("current step"=w217, "enable"=i16 1, "manual"=w244) -> ("Led 8"=→"Led8 2":bool, "Led 10"=→"Led10 2":bool, "Led 11"=→"Led11 2":bool, "Led 7"=→"Led7 2":bool, "Led 1"=→"Led1 2":bool, "Led 6"=→"Led6 2":bool, "Led 2"=→"Led2 2":bool, "Led 12"=→"Led11 3":bool, "Led 5"=→"Led5 2":bool, "Led 4"=→"Led4 2":bool, "Led 3"=→"Led3 2":bool, "Led 9"=→"Led9 2":bool)  [unwired: 1 in]
    n199 = call "MWriteRS232_1.vi"("P3"=w126, "P2"=w127, "P1"=w128, "LAUDA"=w111) -> ()  [unwired: 8 in]
    n200 = Merge Signals(w182, w184, w181) -> (w180:dynamicdata)
    n201 = Boolean To (0,1)(Boolean="Read Seq") -> (0, 1=w129:i16)
    n202 = for {
      N: w129 -> [_]
      tunnel: "Configuration file" -> [w391]
      tunnel: "Read Seq" -> [w390]
      n203 = while {
        tunnel: [w417] -> w413
        tunnel: w391 -> [w416]
        tunnel: w390 -> [w414]
        stop <- w415 stop-if-true
        n204 = call "Read From Measurement File"("Filename"=w416, "Reset"=w414) -> ("Signals"=w417:dynamicdata, "EOF?"=w415:bool)  [unwired: 4 in, 4 out]
      }
      n205 = call "Convert from Dynamic Data"("Dynamic Data Type"=w413) -> ("Array"=w403:dbl[][])  [unwired: 3 in]
      "Config File" <- w403
      n206 = Array Subset(array=w403, index (row)=20 ("index"), length (row)=10 ("length")) -> (w410:dbl[][])  [unwired: 2 in]
      n207 = Array Subset(array=w403, index (row)=10 ("index"), length (row)=10 ("length")) -> (w405:dbl[][])  [unwired: 2 in]
      n208 = Array Subset(array=w403, index (row)=0 ("index"), length (row)=10 ("length")) -> (w404:dbl[][])  [unwired: 2 in]
      n209 = Array Subset(array=w403, index (row)=30 ("index"), length (row)=8 ("length")) -> (w392:dbl[][])  [unwired: 2 in]
      n210 = property on="PumpSeq 4" class="Arr (strict)"("Val(Sgnl)"=w410) -> ()  [unwired: 2 in, 2 out]
      n211 = property on="PumpSeq 2" class="Arr (strict)"("Val(Sgnl)"=w405) -> ()  [unwired: 2 in, 2 out]
      n212 = property on="PumpSeq 3" class="Arr (strict)"("Val(Sgnl)"=w404) -> ()  [unwired: 2 in, 2 out]
      n213 = Index Array(array=w392, index (row)=2, index (col)=0 ("disabled index (col)")) -> ()  [unwired: 1 out]
      n214 = Index Array(array=w392, index (row)=4, index (col)=0 ("disabled index (col)")) -> ()  [unwired: 1 out]
      n215 = Index Array(array=w392, index (row)=0, index (col)=1 ("disabled index (col)")) -> ()  [unwired: 1 out]
      n216 = Index Array(array=w392, index (row)=1, index (col)=1 ("disabled index (col)")) -> ()  [unwired: 1 out]
    }
    n217 = Merge Signals(w179, w180, w36) -> (w71:dynamicdata)
    n218 = call "Build Table"("Include time data"=TRUE, "Signals"=w71) -> ("Table"=w296:string[][])  [unwired: 3 in, 6 out]
    n219 = And(x="?", y="?") -> (x .and. y?=w25:bool)
    n220 = dll-call lib="C:/Users/shresplab/OneDrive - Kemira Oyj/Documents/GitHub/Bertta/BERTTA/x64/Debug/BERTTA.dll" fn="mettler"("port"="Scale port", "msg"=1) -> ("return type"=w18:dbl)  [unwired: 5 in, 2 out]
    n221 = And(x="MASTER CONTROL", y=w25) -> (x .and. y?=w21:bool)
    n222 = Initialize Array(FALSE, 1 ("dimension size")) -> (w23:bool[])
    n223 = Replace Array Subset(array=w23, new element=w21, index=0) -> (w20:bool[])
    n224 = call "Convert to Dynamic Data5"("Double"=w18) -> ("Dynamic Data Type"=→"Waveform Chart 15":dynamicdata)  [unwired: 3 in]
    n225 = Delete From Array(array=w296, length=13, index (col)=0 ("index (row)")) -> (array with subset deleted=→"Table":string[][])  [unwired: 1 in, 1 out]
    n226 = call "DAQ Assistant"("data"=w20, "device name"="PAM Control") -> ()  [unwired: 16 in, 2 out]
    n227 = call "filenameparser_09.vi"("Description"="Description", "start path"="Browse folder", "Project name"="Project name", "User (initials)"="User (initials)", "OK Button in"="OK Button 2") -> ("appended path 2"=w112:path, "appended path"=w292:path)  [unwired: 4 in, 1 out]
    "Output File" <- w112
    n228 = Boolean To (0,1)(Boolean="OK Button") -> (0, 1=w291:i16)
    n229 = for {
      N: w291 -> [_]
      tunnel: w292 -> [w382]
      w386 = " " ("string")
      n230 = property on="Add comment" class="Str"("Val(Sgnl)"="" ("Value (Signaling)")) -> ()  [unwired: 2 in, 2 out]
      n231 = Get Date/Time String(want seconds? (F)=TRUE) -> (date string=w389:string, time string=w387:string)  [unwired: 2 in]
      n232 = Concatenate Strings(w389, w386, w387, w386, "Add comment") -> (w385:string)
      n233 = feedback #9() -> (w384:string[])  [unwired: 1 in]
      n234 = Build Array (concatenate)(w384, w385) -> (w383:string[])
      n235 = feedback-in #9(w383) -> ()
      n236 = Write to Text File(file (use dialog)=w382, text=w383) -> ()  [unwired: 2 in, 3 out]
    }
    n237 = call "Header Names 4.vi"("Dynamic Data"=w71) -> ("Signals Out"=w72:dynamicdata)  [unwired: 10 in]
    n238 = call "Write To Measurement File"("Signals"=w72, "Enable"="OK Button 2", "Filename"=w112) -> ()  [unwired: 14 in, 3 out]
    "Boolean" <- "OK Button 2"
  }
